vi "Wolna czas FVG.vi"(7 "Czas Akcja (Sprawdz)":T1=1 items=["Reset", "Sprawdz"], 8 "error in (no error)":errorcluster, 11 "Zadany":dbl) -> (0 "error out":errorcluster, 2 "Elapsed?":bool)   [LabVIEW 2013]
doc: "Use this template to build a VI to use as a subVI."
uses:
  Kontrolki/FVGs/FVG Czas.ctl
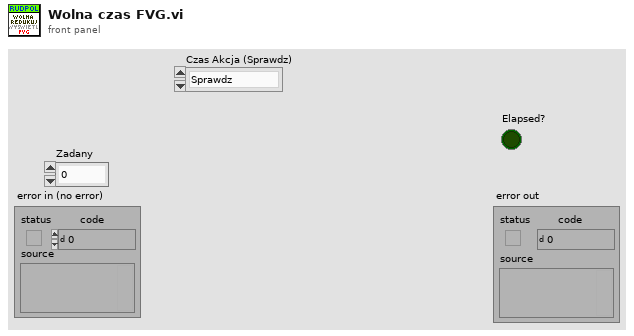
[diagram p1: front panel]
types:
  T1 = typedef "FVG Czas.ctl" = u16
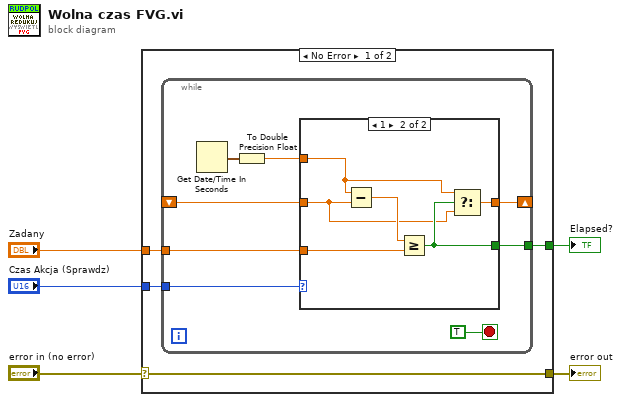
[diagram p0: block diagram]
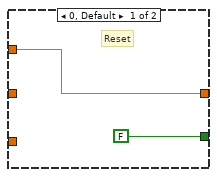
[diagram p2: hidden frame]
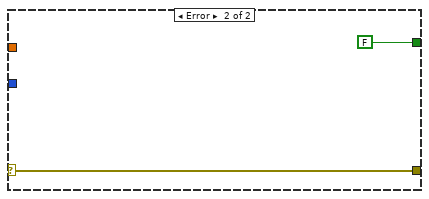
[diagram p3: hidden frame]
diagram:
  n1 = case shown="No Error" "error in (no error)" {
    selector: "error in (no error)" -> [w6 w27]
    tunnel: [w6 w27] -> w4
    tunnel: [w9 FALSE] -> w3
    tunnel: "Czas Akcja (Sprawdz)" -> [w8 _]
    tunnel: "Zadany" -> [w7 _]
    frame No Error {
      n2 = while {
        tunnel: w8 -> [w16]
        shift-right: [w14] -> _
        shift-left: _ -> [w11]
        tunnel: w7 -> [w15]
        tunnel: [w10] -> w9
        stop <- TRUE stop-if-true
        n3 = Get Date/Time In Seconds() -> (seconds since 1Jan1904=w13:timestamp)
        n4 = To Double Precision Float(number=w13) -> (double precision float=w12:dbl)
        n5 = case shown="1" w16 {
          tunnel: w15 -> [_ w25]
          tunnel: [w19 w20] -> w14
          tunnel: w12 -> [w19 w21]
          tunnel: w11 -> [_ w22]
          tunnel: [FALSE w23] -> w10
          frame 0, Default {
            # "Reset"
          }
          frame 1 {
            n6 = Subtract(x=w21, y=w22) -> (x-y=w24:dbl)
            n7 = Greater Or Equal?(x=w24, y=w25) -> (x >= y?=w23:bool)
            n8 = Select(t=w21, s=w23, f=w22) -> (s? t:f=w20:dbl)
          }
        }
      }
    }
    frame Error {
    }
  }
  "error out" <- w4
  "Elapsed?" <- w3
